vi "Set Allow Debugging for VIs in Folder.vi"(8 "error in (no error)":errorcluster, 10 "Allow Debugging?":bool, 11 "VI Folder":path) -> (0 "error out":errorcluster, 3 "VI List":path[](array[path]))   [LabVIEW 2016, in "SLL Scripting.lvlib"]
doc: "This is used to set/unset the \"Allow Debugging\" option for all VIs in the specified folder."
uses:
  SLL Scripting.lvlib
panel:
  out "Progress":i32
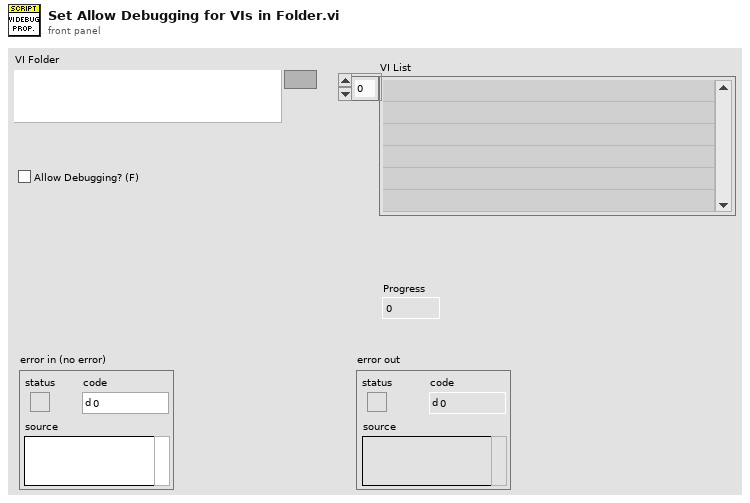
[diagram p1: front panel]
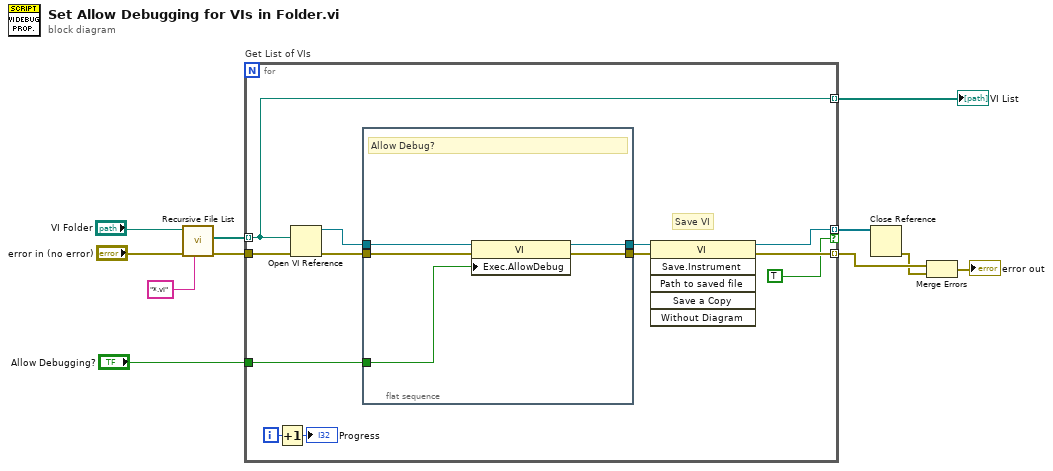
[diagram p0: block diagram]
diagram:
  n1 = call <vilib>:"Recursive File List.vi"("pattern"="*.vi", "error in (no error)"="error in (no error)", "Folder Path"="VI Folder") -> ("error out"=w5:errorcluster, "All Files in Dir"=w8:path[])  [unwired: 4 in, 3 out]
  n2 = for "Get List of VIs" {
    tunnel: [w21] -> w11 mode=indexing if=TRUE
    tunnel: w8 -> [w18] mode=indexing
    tunnel: [w18] -> w7 mode=indexing
    tunnel: w5 -> [w20]
    tunnel: [w22] -> w4 mode=indexing
    tunnel: "Allow Debugging?" -> [w17]
    i -> [w23]
    # "Save VI"
    n3 = Increment(x=w23) -> (x+1=→"Progress":i32)
    n4 = Open VI Reference(vi path=w18, error in (no error)=w20) -> (vi reference=w16:refnum<vi>, error out=w15:errorcluster)  [unwired: 4 in]
    n5 = flat-sequence {
      tunnel: w16 -> [w26]
      tunnel: w15 -> [w28]
      tunnel: [w27] -> w14
      tunnel: [w25] -> w13
      tunnel: w17 -> [w24]
      frame #0 {
        # "Allow Debug?"
        n6 = property class="VI"(reference=w26, error in=w28, "Exec.AllowDebug"=w24) -> (reference out=w25:refnum<vi>, error out=w27:errorcluster)
      }
    }
    n7 = invoke class="VI" method="Save.Instrument"(reference=w13, error in=w14) -> (reference out=w21:refnum<vi>, error out=w22:errorcluster)  [unwired: 4 in, 4 out]
  }
  "VI List" <- w7
  n8 = Close Reference(reference=w11) -> (error out=w3:errorcluster)  [unwired: 1 in]
  n9 = Merge Errors(w4, w3) -> (→"error out":errorcluster)
